vi "Select Two Distinct Cut Indices in Ascending Order.vi"(11 "Schedule":u16[](array[numeric])) -> (2 "Index 2":i32, 3 "Index 1":i32)   [LabVIEW 2013, in "GA.lvclass"]
uses:
  GA.lvclass
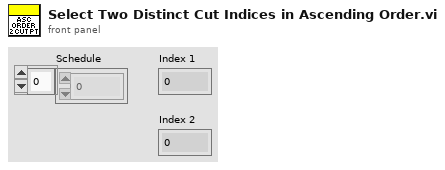
[diagram p1: front panel]
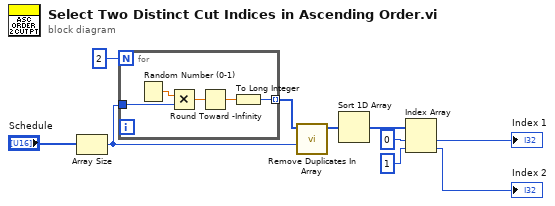
[diagram p0: block diagram]
diagram:
  n1 = Array Size(array="Schedule") -> (size(s)=w6:i32)
  n2 = for {
    N: 2 -> [_]
    tunnel: w6 -> [w12]
    tunnel: [w11] -> w7 mode=indexing
    n3 = Random Number (0-1)() -> (number: 0 to 1=w15:dbl)
    n4 = Multiply(x=w15, y=w12) -> (x*y=w14:dbl)
    n5 = Round Toward -Infinity(1:w14) -> (0:w13:dbl)
    n6 = To Long Integer(number=w13) -> (32bit integer=w11:i32)
  }
  n7 = call "Remove Duplicates In Array.vi"("Max Index Bound"=w6, "Random Numbers Array"=w7) -> ("Random Numbers Array without Duplicates"=w2:i32[])  [unwired: 9 in]
  n8 = Sort 1D Array(array=w2) -> (sorted array=w1:i32[])
  n9 = Index Array(array=w1, index #1=0 ("index"), index #2=1 ("index")) -> (element #1=→"Index 1":i32, element #2=→"Index 2":i32)
